vi "ActionVIOnLoad.vi"(8 "error in":errorcluster, 11 "custom device ref":T1 format="%.0x") -> (0 "error out":errorcluster, 3 "custom device ref out":T1 format="%.0x")   [LabVIEW 2020, in "AIM ARINC 429 System Explorer.lvlib" / "Implementation.lvlib"]
uses:
  Implementation.lvlib
  Scripting/AIM/AIM ARINC 429 Scripting.lvlib
  <vilib>/NI VeriStand/Custom Device Tools/Custom Device Utility Library/Custom Device Utility Library.lvlib
  Scripting/AIM/Constants.vi
  <vilib>/NI VeriStand/Custom Device Tools/Custom Device Utility Library/NI VeriStand - Search for Item by GUID.vi
  <vilib>/NI VeriStand/Custom Device API/Custom Device Item Ref.ctl
  <vilib>/NI VeriStand/Custom Device API/Custom Device API.lvlib
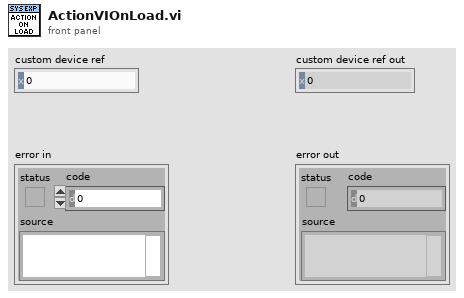
[diagram p1: front panel]
types:
  T1 = typedef "Custom Device API.lvlib/Custom Device Item Ref.ctl" = u64
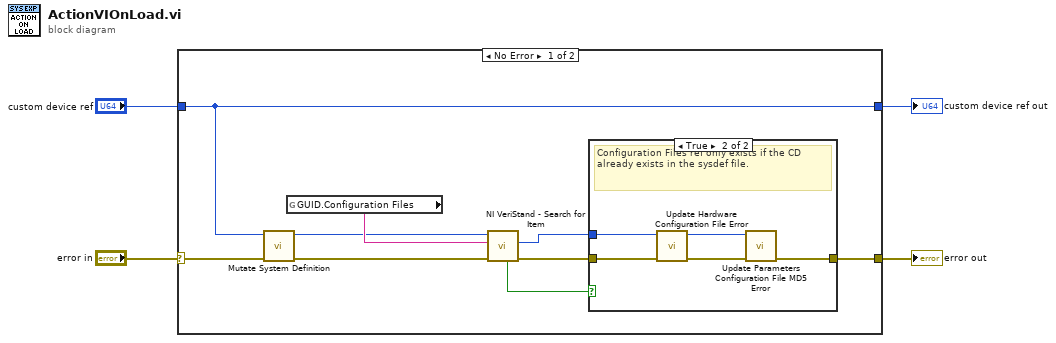
[diagram p0: block diagram]
diagram:
  n1 = case shown="No Error" "error in" {
    selector: "error in" -> [w13 w20]
    tunnel: "custom device ref" -> [w6 w21]
    tunnel: [w6 w21] -> w2
    tunnel: [w10 w20] -> w1
    frame No Error {
      n2 = call "Mutate System Definition.vi"("error in (no error)"=w13, "Device Ref in"=w6) -> ("error out"=w7:errorcluster, "Device Ref out"=w5:T1)  [unwired: 8 in]
      n3 = global read "Constants.vi" "GUID.Configuration Files"() -> (w11:string)
      n4 = call-poly <vilib>:"NI VeriStand - Search for Item.vi"("error in"=w7, "Item GUID"=w11, "Section Ref in"=w5) -> ("error out"=w12:errorcluster, "Item Ref"=w9:T1, "Found"=w8:bool)  [unwired: 5 in, 1 out]
      n5 = case shown="True" w8 {
        tunnel: w12 -> [w14 w19]
        tunnel: [w14 w16] -> w10
        tunnel: w9 -> [_ w18]
        frame False {
          # "Expected when a new CD is created."
        }
        frame True {
          # "Configuration Files ref only exists if the CD already exists in the sysdef file."
          n6 = call "Update Hardware Configuration File Error.vi"("error in"=w19, "Configuration files Ref"=w18) -> ("error out"=w17:errorcluster, "Configuration files Ref out"=w15:T1)  [unwired: 8 in]
          n7 = call "Update Parameters Configuration File MD5 Error.vi"("error in"=w17, "configuration files ref"=w15) -> ("error out"=w16:errorcluster)  [unwired: 8 in, 1 out]
        }
      }
    }
    frame Error {
    }
  }
  "error out" <- w1
  "custom device ref out" <- w2
